vi "Search ROM.vi"(7 "1-Wire DIO Pin":refnum<k21>="ConnectorA/DIO15", 8 "Error In":errorcluster) -> (0 "Error Out":errorcluster, 1 "LastDeviceFlag":bool, 2 "ROM Array":u64[](array[numeric]) format="%x")   [LabVIEW 2014, in "Maxim 1-Wire.lvlib"]
doc: "SEARCH ROM [F0h]\nWhen a system is initially powered up, the master must identify the ROM codes of all slave devices on the bus, which allows the master to determine the number of slaves and their device types. The master learns the ROM codes through a process of elimination that requires the master to perform a Search ROM cycle (i.e., Search ROM command followed by data exchange) as many times as necessary to identify all of the slave devices. If there is only one slave on the bus, the simpler Read ROM command (see below) can be used in place of the Search ROM process. For a detailed explanation of the Search ROM procedure, refer to the iButton® Book of Standards at www.maxim-ic.com/ibuttonbook. After every Search ROM cycle, the bus master must return to Step 1 (Initialization) in the transaction sequence."
uses:
  Maxim 1-Wire.lvlib
  Search ROM Variables.ctl
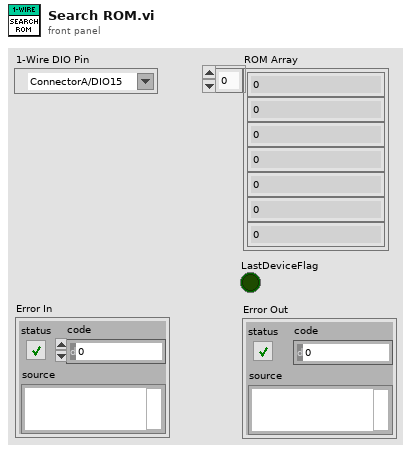
[diagram p1: front panel]
types:
  T1 = typedef "Maxim 1-Wire.lvlib/Search ROM Variables.ctl" = cluster{"id_bit_number":i16, "comp_id_bit":bool, "id_bit":bool, "LastDeviceFlag":bool, "LastDiscrepancy":i16, "LastFamilyDiscrepancy":i16, "last_zero":i16, "ROM_NO":u64, "search_direction":bool}
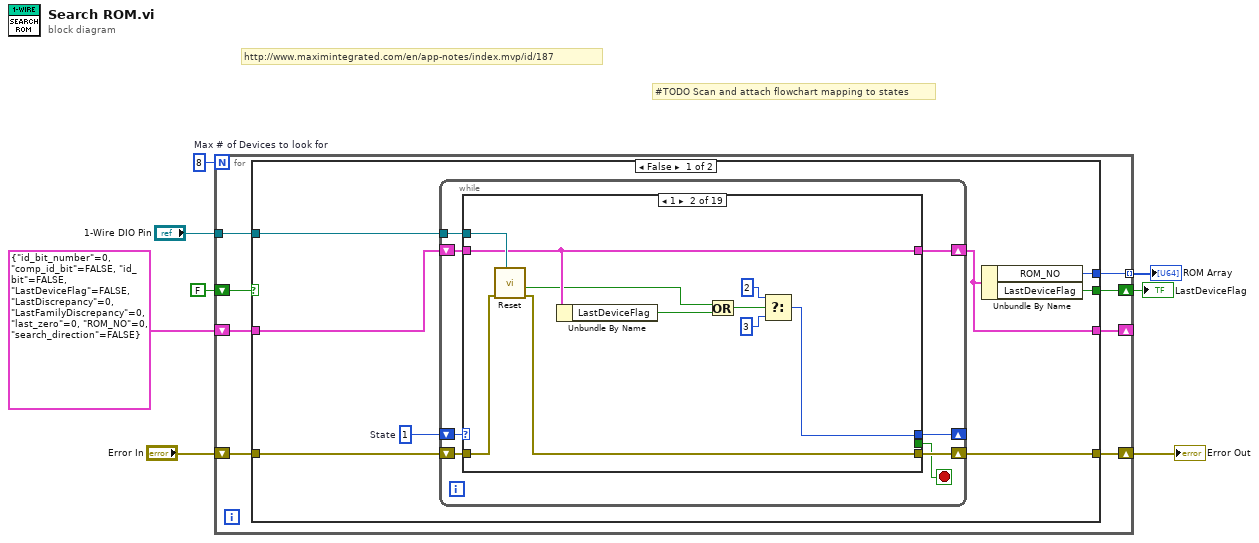
[diagram p0: block diagram]
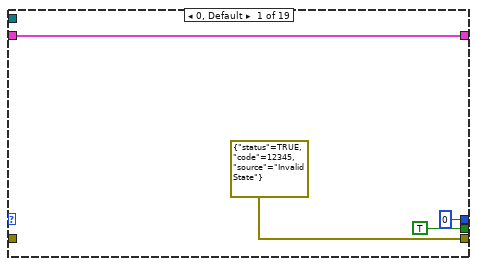
[diagram p2: hidden frame]
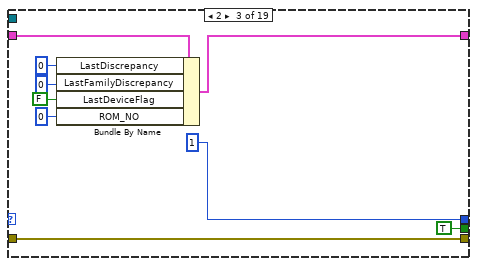
[diagram p3: hidden frame]
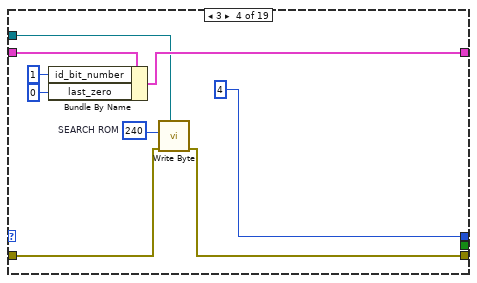
[diagram p4: hidden frame]
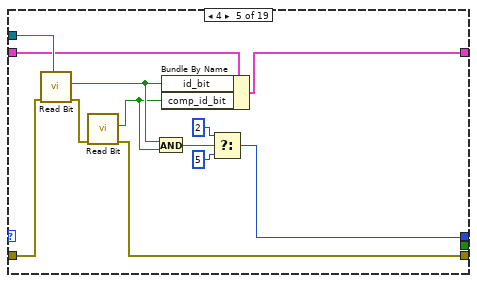
[diagram p5: hidden frame]
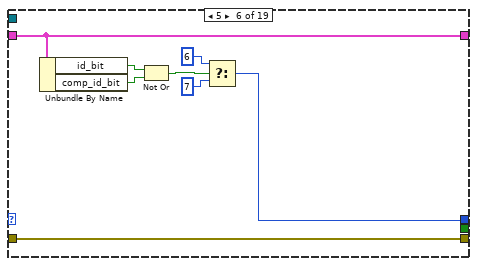
[diagram p6: hidden frame]
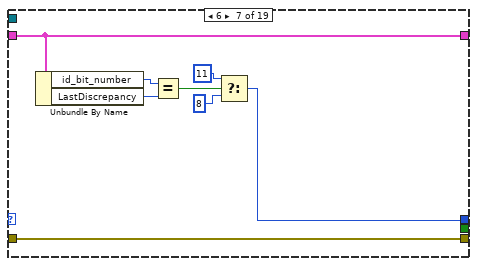
[diagram p7: hidden frame]
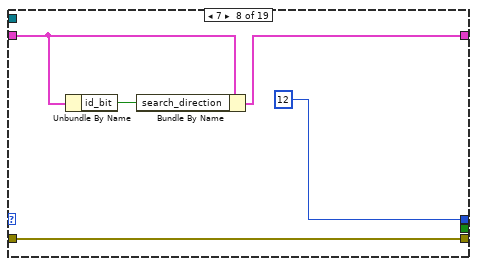
[diagram p8: hidden frame]
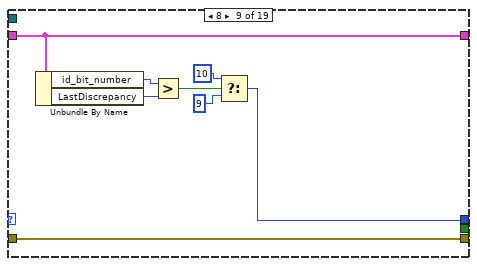
[diagram p9: hidden frame]
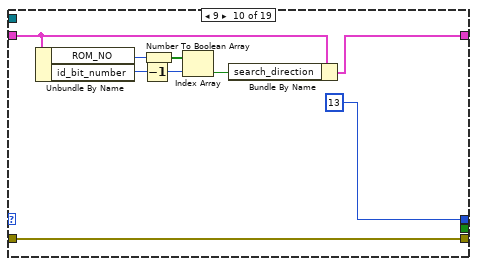
[diagram p10: hidden frame]
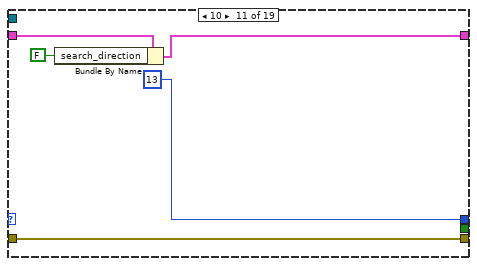
[diagram p11: hidden frame]
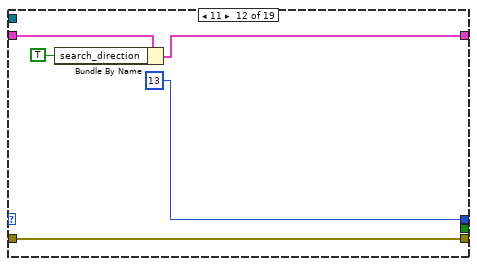
[diagram p12: hidden frame]
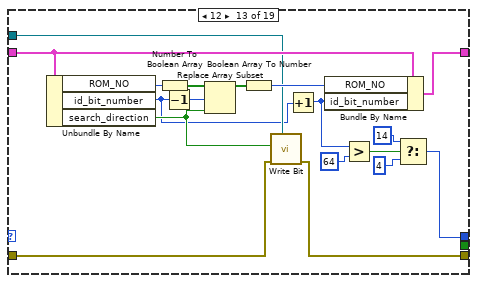
[diagram p13: hidden frame]
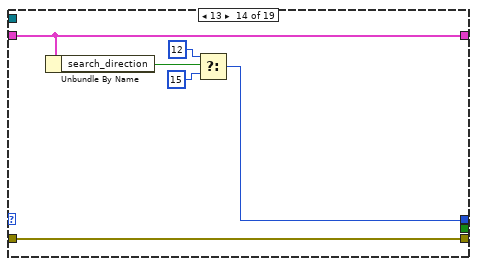
[diagram p14: hidden frame]
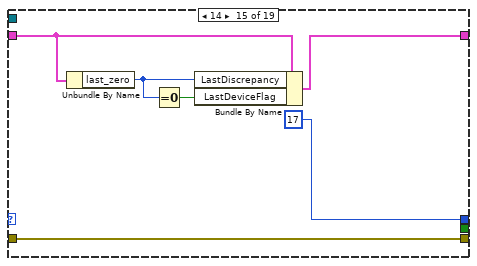
[diagram p15: hidden frame]
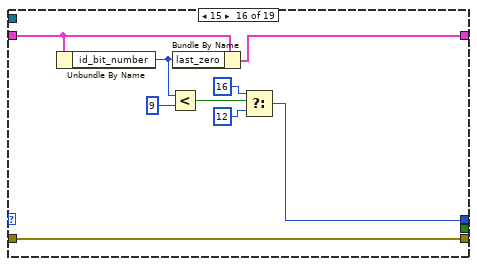
[diagram p16: hidden frame]
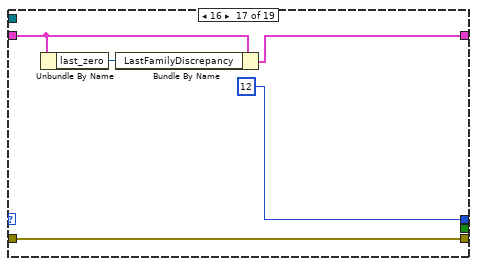
[diagram p17: hidden frame]
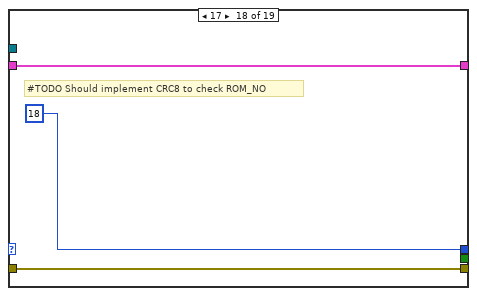
[diagram p18: hidden frame]
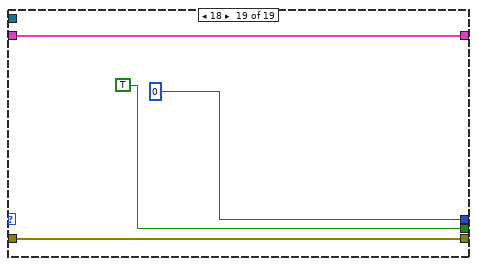
[diagram p19: hidden frame]
diagram:
  w4 = 8  # Max # of Devices to look for
  # "#TODO Scan and attach flowchart mapping to states"
  # "http://www.maximintegrated.com/en/app-notes/index.mvp/id/187"
  n1 = for {
    N: w4 -> [_]
    tunnel: "1-Wire DIO Pin" -> [w16]
    shift-right: [w14] -> w6
    shift-left: "Error In" -> [w15]
    tunnel: [w13] -> w5 mode=indexing
    shift-right: [w12] -> w1
    shift-left: FALSE ("LastDeviceFlag") -> [w11]
    shift-right: [w9] -> _
    shift-left: T1 {"id_bit_number"=0, "comp_id_bit"=FALSE, "id_bit"=FALSE, "LastDeviceFlag"=FALSE, "LastDiscrepancy"=0, "LastFamilyDiscrepancy"=0, "last_zero"=0, "ROM_NO"=0, "search_direction"=FALSE} ("Cluster") -> [w10]
    n2 = case shown="False" w11 {
      selector: w11 -> [_ w177]
      tunnel: w16 -> [w23 _]
      tunnel: w15 -> [w22 w178]
      tunnel: [w21 w178] -> w14
      tunnel: [w20 _] -> w13
      tunnel: [w19 w177] -> w12
      tunnel: w10 -> [w18 w176]
      tunnel: [w17 w176] -> w9
      frame False {
        w24 = i16 1  # State
        n3 = while {
          shift-right: [w30] -> w17
          shift-left: w18 -> [w29]
          shift-right: [w27] -> w21
          shift-left: w22 -> [w28]
          shift-right: [w26] -> _
          shift-left: w24 -> [w32]
          tunnel: w23 -> [w31]
          stop <- w25 stop-if-true
          n4 = case shown="1" w32 {
            tunnel: w31 -> [_ w46 _ w59 w75 _ _ _ _ _ _ _ w136 _ _ _ _ _ _]
            tunnel: [w36 w43 w53 w61 w71 w83 w91 w94 w104 w107 w117 w122 w139 w147 w153 w161 w166 w171 w175] -> w30
            tunnel: w29 -> [w36 w43 w54 w62 w72 w83 w91 w95 w104 w108 w118 w123 w140 w147 w152 w162 w167 w171 w175]
            tunnel: w28 -> [_ w45 w55 w58 w74 w84 w92 w97 w105 w114 w119 w124 w134 w148 w154 w163 w168 w170 w174]
            tunnel: [errorcluster {"status"=TRUE, "code"=12345, "source"="Invalid State"} ("Error In") w44 w55 w57 w73 w84 w92 w97 w105 w114 w119 w124 w133 w148 w154 w163 w168 w170 w174] -> w27
            tunnel: [i16 0 ("State") w38 i16 1 ("State") i16 4 ("y") w65 w77 w85 i16 12 ("State") w98 i16 13 ("State") i16 13 ("State") i16 13 ("State") w125 w143 i16 17 ("State") w155 i16 12 ("State") i16 18 ("State") i16 0 ("State")] -> w26
            tunnel: [TRUE _ TRUE _ _ _ _ _ _ _ _ _ _ _ _ _ _ _ TRUE] -> w25
            frame 0, Default {
            }
            frame 1 {
              n5 = call "Reset.vi"("1-Wire DIO Pin"=w46, "error in"=w45) -> ("error out"=w44:errorcluster, "0 = Device Present / 1=no"=w42:bool)  [unwired: 8 in]
              n6 = Unbundle By Name(w43) -> ("LastDeviceFlag"=w37:bool)
              n7 = Or(x=w42, y=w37) -> (x .or. y?=w41:bool)
              n8 = Select(t=i16 2 ("y"), s=w41, f=i16 3 ("y")) -> (s? t:f=w38:i16)
            }
            frame 2 {
              n9 = Bundle By Name(cluster=w54, "LastDiscrepancy"=i16 0, "LastFamilyDiscrepancy"=i16 0, "LastDeviceFlag"=FALSE, "ROM_NO"=u64 0) -> (w53:T1)
            }
            frame 3 {
              w60 = u8 240  # SEARCH ROM
              n10 = Bundle By Name(cluster=w62, "id_bit_number"=i16 1, "last_zero"=i16 0) -> (w61:T1)
              n11 = call "Write Byte.vi"("1-Wire DIO Pin"=w59, "error in"=w58, "Tx data"=w60) -> ("error out"=w57:errorcluster)  [unwired: 8 in]
            }
            frame 4 {
              n12 = call "Read Bit.vi"("1-Wire DIO Pin"=w75, "error in"=w74) -> ("error out"=w76:errorcluster, "Bit Read"=w70:bool)  [unwired: 8 in]
              n13 = call "Read Bit.vi"("error in"=w76) -> ("error out"=w73:errorcluster, "Bit Read"=w69:bool)  [unwired: 9 in]
              n14 = And(x=w70, y=w69) -> (x .and. y?=w68:bool)
              n15 = Bundle By Name(cluster=w72, "id_bit"=w70, "comp_id_bit"=w69) -> (w71:T1)
              n16 = Select(t=i16 2 ("State"), s=w68, f=i16 5 ("State")) -> (s? t:f=w65:i16)
            }
            frame 5 {
              n17 = Unbundle By Name(w83) -> ("id_bit"=w81:bool, "comp_id_bit"=w82:bool)
              n18 = Not Or(1:w82, 2:w81) -> (0:w78:bool)
              n19 = Select(t=i16 6 ("State"), s=w78, f=i16 7 ("State")) -> (s? t:f=w77:i16)
            }
            frame 6 {
              n20 = Unbundle By Name(w91) -> ("id_bit_number"=w89:i16, "LastDiscrepancy"=w90:i16)
              n21 = Equal?(x=w89, y=w90) -> (x = y?=w86:bool)
              n22 = Select(t=i16 11 ("State"), s=w86, f=i16 8 ("State")) -> (s? t:f=w85:i16)
            }
            frame 7 {
              n23 = Unbundle By Name(w95) -> ("id_bit"=w96:bool)
              n24 = Bundle By Name(cluster=w95, "search_direction"=w96) -> (w94:T1)
            }
            frame 8 {
              n25 = Unbundle By Name(w104) -> ("id_bit_number"=w102:i16, "LastDiscrepancy"=w103:i16)
              n26 = Greater?(x=w102, y=w103) -> (0:w99:bool)
              n27 = Select(t=i16 10 ("State"), s=w99, f=i16 9 ("State")) -> (s? t:f=w98:i16)
            }
            frame 9 {
              n28 = Unbundle By Name(w108) -> ("ROM_NO"=w112:u64, "id_bit_number"=w111:i16)
              n29 = Decrement(x=w111) -> (x-1=w110:i16)
              n30 = Number To Boolean Array(number=w112) -> (Boolean array=w113:bool[])
              n31 = Index Array(array=w113, index=w110) -> (element=w109:bool)
              n32 = Bundle By Name(cluster=w108, "search_direction"=w109) -> (w107:T1)
            }
            frame 10 {
              n33 = Bundle By Name(cluster=w118, "search_direction"=FALSE) -> (w117:T1)
            }
            frame 11 {
              n34 = Bundle By Name(cluster=w123, "search_direction"=TRUE) -> (w122:T1)
            }
            frame 12 {
              n35 = Unbundle By Name(w140) -> ("ROM_NO"=w141:u64, "id_bit_number"=w127:i16, "search_direction"=w135:bool)
              n36 = Number To Boolean Array(number=w141) -> (Boolean array=w142:bool[])
              n37 = Decrement(x=w127) -> (x-1=w132:i16)
              n38 = Replace Array Subset(array=w142, new element=w135, index=w132) -> (w137:bool[])
              n39 = Boolean Array To Number(Boolean array=w137) -> (number=w138:u64)
              n40 = call "Write Bit.vi"("1-Wire DIO Pin"=w136, "Error In"=w134, "Bit"=w135) -> ("Error Out"=w133:errorcluster)  [unwired: 8 in]
              n41 = Increment(x=w127) -> (x+1=w128:i16)
              n42 = Bundle By Name(cluster=w140, "ROM_NO"=w138, "id_bit_number"=w128) -> (w139:T1)
              n43 = Greater?(x=w128, y=i16 64) -> (0:w129:bool)
              n44 = Select(t=i16 14 ("State"), s=w129, f=i16 4 ("State")) -> (s? t:f=w125:i16)
            }
            frame 13 {
              n45 = Unbundle By Name(w147) -> ("search_direction"=w144:bool)
              n46 = Select(t=i16 12 ("State"), s=w144, f=i16 15 ("State")) -> (s? t:f=w143:i16)
            }
            frame 14 {
              n47 = Unbundle By Name(w152) -> ("last_zero"=w151:i16)
              n48 = Equal To 0?(x=w151) -> (x = 0?=w150:bool)
              n49 = Bundle By Name(cluster=w152, "LastDiscrepancy"=w151, "LastDeviceFlag"=w150) -> (w153:T1)
            }
            frame 15 {
              n50 = Unbundle By Name(w162) -> ("id_bit_number"=w160:i16)
              n51 = Less?(x=w160, y=i16 9) -> (x < y?=w156:bool)
              n52 = Bundle By Name(cluster=w162, "last_zero"=w160) -> (w161:T1)
              n53 = Select(t=i16 16 ("State"), s=w156, f=i16 12 ("State")) -> (s? t:f=w155:i16)
            }
            frame 16 {
              n54 = Unbundle By Name(w167) -> ("last_zero"=w165:i16)
              n55 = Bundle By Name(cluster=w167, "LastFamilyDiscrepancy"=w165) -> (w166:T1)
            }
            frame 17 {
              # "#TODO Should implement CRC8 to check ROM_NO"
            }
            frame 18 {
            }
          }
        }
        n56 = Unbundle By Name(w17) -> ("ROM_NO"=w20:u64, "LastDeviceFlag"=w19:bool)
      }
      frame True {
      }
    }
  }
  "Error Out" <- w6
  "ROM Array" <- w5
  "LastDeviceFlag" <- w1
